vi "StopClone.vi"(8 "error in (no error)":errorcluster, 9 "Wait for Module to stop?":bool, 11 "ModuleAdmin":refnum<class "ModuleAdmin.lvclass">) -> (0 "error out":errorcluster)   [LabVIEW 2018, in "SensorShared.lvlib"]
doc: "This VI sends a message to a sensor clone to stop any action that it is currently taking."
uses:
  SensorShared.lvlib
  <userlib>/NIST/ModuleAdminLib/ModuleAdmin/ModuleAdmin.lvclass
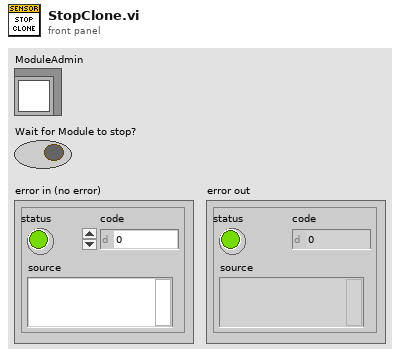
[diagram p1: front panel]
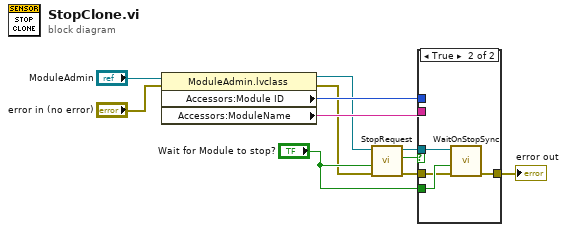
[diagram p0: block diagram]
diagram:
  n1 = property class="ModuleAdmin.lvclass"(reference="ModuleAdmin", error in="error in (no error)") -> (reference out=w5:refnum<class "ModuleAdmin.lvclass">, error out=w3:errorcluster, "Accessors:Module ID"=w8:i32, "Accessors:ModuleName"=w7:string)
  n2 = call "StopRequest.vi"("error in (no error)"=w3, "Wait for Module to stop? (F)"="Wait for Module to stop?", "ModuleAdminIn"=w5) -> ("error out"=w9:errorcluster, "Stop Request Sent"=w10:bool, "ModuleAdminOut"=w1:refnum<class "ModuleAdmin.lvclass">)  [unwired: 6 in]
  n3 = case shown="True" w10 {
    tunnel: w8 -> [_ _]
    tunnel: w7 -> [_ _]
    tunnel: "Wait for Module to stop?" -> [_ w16]
    tunnel: [w12 w15] -> w2
    tunnel: w9 -> [w12 w14]
    tunnel: w1 -> [_ w13]
    frame False {
    }
    frame True {
      n4 = call <userlib>:"WaitOnStopSync.vi"("error in (no error)"=w14, "WaitForModuleToStop?"=w16, "ModuleAdmin"=w13) -> ("error out"=w15:errorcluster)  [unwired: 7 in, 1 out]
    }
  }
  "error out" <- w2
